vi "ControlProcessWindow.vi"(0 "reference in":refnum<class "Active object Event.lvclass">, 2 "ShowProcessWindow":bool, 5 "error in (no error)":errorcluster) -> (14 "reference out":refnum<class "Active object Event.lvclass">, 19 "error out":errorcluster)   [LabVIEW 2019, in "Active object Event.lvclass"]
uses:
  Active object Event.lvclass
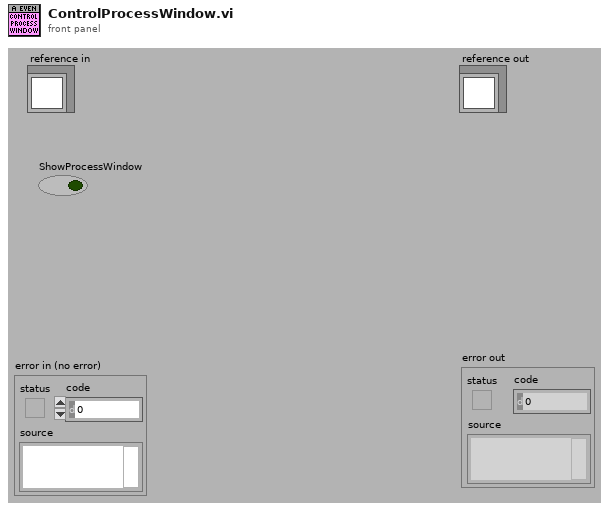
[diagram p1: front panel]
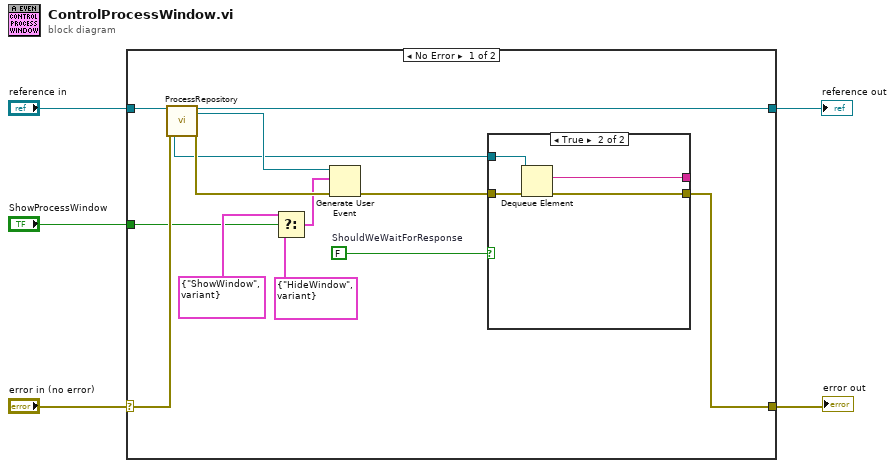
[diagram p0: block diagram]
diagram:
  n1 = case shown="No Error" "error in (no error)" {
    selector: "error in (no error)" -> [w18 w25]
    tunnel: [w11 w25] -> w4
    tunnel: [w16 w24] -> w2
    tunnel: "reference in" -> [w17 w24]
    tunnel: "ShowProcessWindow" -> [w7 _]
    frame No Error {
      w14 = FALSE  # ShouldWeWaitForResponse
      n2 = call "ProcessRepository.vi"("reference in"=w17, "error in (no error)"=w18) -> ("QueueFromProcess"=w10:refnum<queue>, "reference out"=w16:refnum<class "Active object Event.lvclass">, "EventsToProcess"=w15:refnum<user-event>, "error out"=w12:errorcluster)  [unwired: 10 in, 4 out]
      n3 = Select(t=cluster{"Command":string, "Data":variant} {"Command"="ShowWindow", "Data"=variant} ("MessageToProcess"), s=w7, f=cluster{"Command":string, "Data":variant} {"Command"="HideWindow", "Data"=variant} ("MessageToProcess")) -> (s? t:f=w6:cluster{"Command":string, "Data":variant})
      n4 = Generate User Event(user event=w15, event data cluster=w6, error in=w12) -> (error out=w13:errorcluster)  [unwired: 1 in, 1 out]
      n5 = case shown="True" w14 {
        tunnel: w13 -> [w19 w23]
        tunnel: [_ w22] -> _
        tunnel: [w19 w21] -> w11
        tunnel: w10 -> [_ w20]
        frame False {
        }
        frame True {
          n6 = Dequeue Element(queue=w20, error in (no error)=w23) -> (element=w22:string, error out=w21:errorcluster)  [unwired: 1 in, 2 out]
        }
      }
    }
    frame Error {
    }
  }
  "error out" <- w4
  "reference out" <- w2
